vi "SbigOpen.vi"(2 "SbigDataList":cluster{"TagName":string, "Serial":string}[](array[cluster])=[{"TagName"="PI1-SBIG", "Serial"="01082913E_"}, {"TagName"="PI2-SBIG", "Serial"="02083139__"}], 9 "error in":errorcluster) -> (0 "Sbig Names out":string[](array[string])=["PI1-SBIG", "PI2-SBIG"], 6 "error out":errorcluster, 7 "Sbig infos":T1[](array[typedef])=[{"Readout modes number"=10, "Readout modes"=[{"Width"=765, "Height"=510, "Gain"=2.63, "pixelWidth"=9.0, "pixelHeight"=9.0}, {"Width"=382, "Height"=255, "Gain"=2.63, "pixelWidth"=18.0, "pixelHeight"=18.0}, {"Width"=255, "Height"=170, "Gain"=2.63, "pixelWidth"=27.0, "pixelHeight"=27.0}, {"Width"=765, "Height"=0, "Gain"=2.63, "pixelWidth"=9.0, "pixelHeight"=9.0}, {"Width"=382, "Height"=0, "Gain"=2.63, "pixelWidth"=18.0, "pixelHeight"=9.0}, {"Width"=255, "Height"=0, "Gain"=2.63, "pixelWidth"=27.0, "pixelHeight"=9.0}, {"Width"=765, "Height"=510, "Gain"=2.63, "pixelWidth"=9.0, "pixelHeight"=9.0}, {"Width"=382, "Height"=255, "Gain"=2.63, "pixelWidth"=18.0, "pixelHeight"=18.0}, {"Width"=255, "Height"=170, "Gain"=2.63, "pixelWidth"=27.0, "pixelHeight"=27.0}, {"Width"=85, "Height"=56, "Gain"=2.63, "pixelWidth"=81.0, "pixelHeight"=81.0}], "Handle"=[2]}, {"Readout modes number"=0, "Readout modes"=[], "Handle"=[]}])   [LabVIEW 2009]
uses:
  Controls/SbigReference.ctl
panel:
  out "Sbigs":string[](array[string])
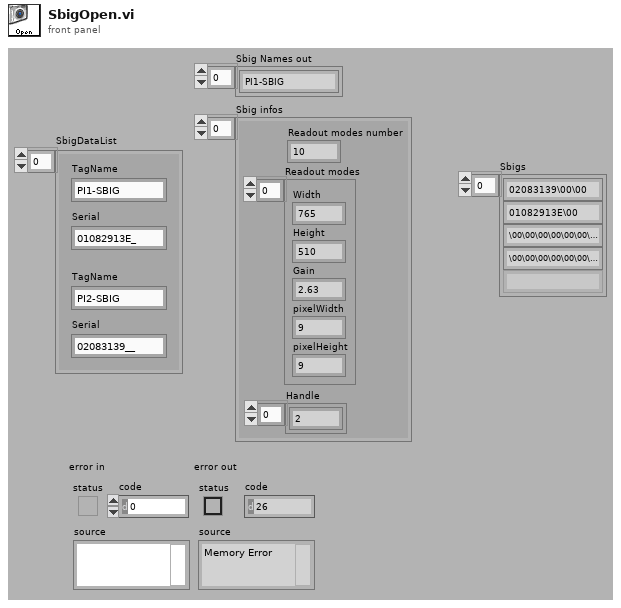
[diagram p1: front panel]
types:
  T1 = typedef "SbigReference.ctl" = cluster{"Readout modes number":u16, "Readout modes":cluster{"Width":u16, "Height":u16, "Gain":dbl, "pixelWidth":dbl, "pixelHeight":dbl}[], "Handle":u16[]}
  T2 = enum16{"0-NoCommand", "1-StartExposure", "2-EndExposure", "3-ReadoutLine", "4-DumpLines", "5-SetTemperatureRegulation", "6-QueryTemperatureStatus", "7-ActivateRelay", "8-PulseOut", "9-EstablishLink", "10-GetDriverInfo", "11-GetCCDInfo", "12-QueryCommandStatus", "13-MiscellaneousControl", "14-ReadSubstractLine", "15-UpdateClock", "16-ReadOffset", "17-OpenDriver", "18-CloseDriver", "19-TXSerialBytes", "20-GetSerialStatus", "21-AOTipTilt", "22-AOSetFocus", "23-AODelay", "24-GetTurboStatus", "25-EndReadout", "26-GetUSTimer", "27-OpenDevice", "28-CloseDevice", "29-SetIRQL", "30-GetIRQL", "31-GetLine", "32-GetLinkStatus", "33-GetDriverHandle", "34-SetDriverHandle", "35-StartReadout", "36-GetErrorString", "37-SetDriverControl", "38-GetDriverControl", "39-USBADControl", "40-QueryUSB", "41-GetPentiumCycleCount", "42-RWUSBI2C", "43-CFW"}
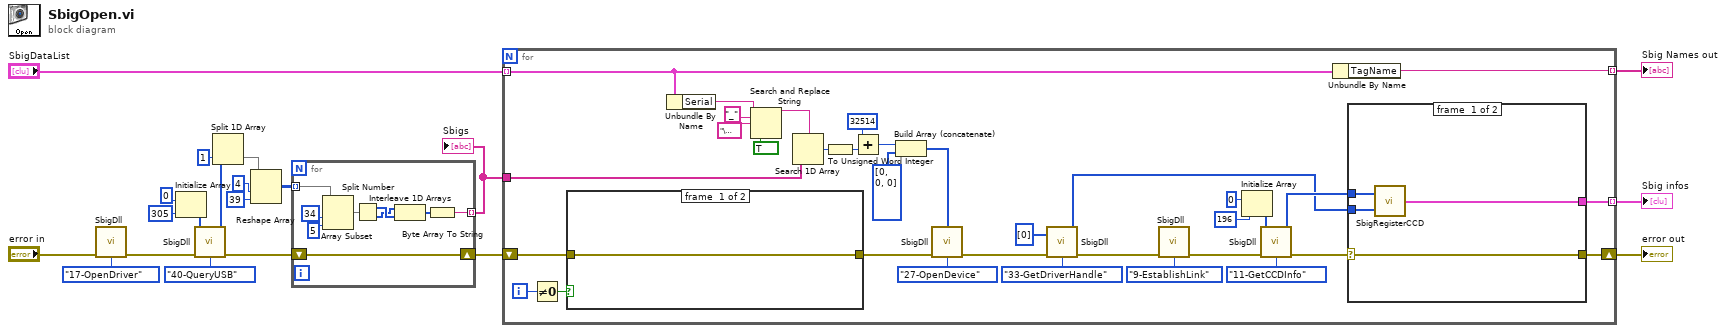
[diagram p0: block diagram]
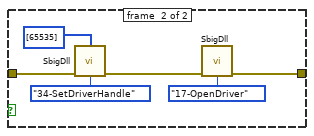
[diagram p2: hidden frame]
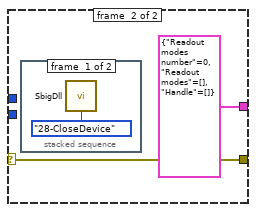
[diagram p3: hidden frame]
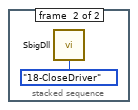
[diagram p4: hidden frame]
diagram:
  n1 = call "SbigDll.vi"("error in (no error)"="error in", "Command"=T2."17-OpenDriver") -> ("error out"=w6:errorcluster)  [unwired: 2 in, 3 out]
  n2 = Initialize Array(u16 0, 305 ("taille de la dimension")) -> (w5:u16[])
  n3 = call "SbigDll.vi"("error in (no error)"=w6, "Command"=T2."40-QueryUSB", "Results In"=w5) -> ("error out"=w15:errorcluster, "Results Out"=w13:u16[])  [unwired: 1 in, 2 out]
  n4 = Split 1D Array(array=w13, index=1 ("indice")) -> (second subarray=w14:u16[])  [unwired: 1 out]
  n5 = Reshape Array(w14, 4 ("taille de la dimension"), 39 ("taille de la dimension")) -> (w4:u16[][])
  n6 = for {
    shift-right: [w27] -> w3
    shift-left: w15 -> [w27]
    tunnel: [w28] -> w2 mode=indexing
    tunnel: w4 -> [w21] mode=indexing
    n7 = Array Subset(array=w21, index=34 ("indice"), length=5 ("longueur")) -> (w22:u16[])
    n8 = Split Number(x=w22) -> (hi(x)=w24:u8[], lo(x)=w23:u8[])
    n9 = Interleave 1D Arrays(w23, w24) -> (w29:u8[])
    n10 = Byte Array To String(unsigned byte array=w29) -> (string=w28:string)
  }
  "Sbigs" <- w2
  n11 = for {
    shift-right: [w53] -> w20
    shift-left: w3 -> [w36]
    tunnel: "SbigDataList" -> [w50] mode=indexing
    tunnel: [w52] -> w17 mode=indexing
    tunnel: [w49] -> w18 mode=indexing
    tunnel: w2 -> [w48]
    i -> [w38]
    n12 = Not Equal To 0?(x=w38) -> (x != 0?=w37:bool)
    n13 = case shown="True" w37 {
      tunnel: w36 -> [w64 w69]
      tunnel: [w64 w65] -> w35
      frame #0 {
      }
      frame #1 {
        n14 = call "SbigDll.vi"("error in (no error)"=w69, "Command"=T2."34-SetDriverHandle", "Parameters"=u16[] [65535] ("Results In")) -> ("error out"=w66:errorcluster)  [unwired: 1 in, 3 out]
        n15 = call "SbigDll.vi"("error in (no error)"=w66, "Command"=T2."17-OpenDriver") -> ("error out"=w65:errorcluster)  [unwired: 2 in, 3 out]
      }
    }
    n16 = Unbundle By Name(w50) -> ("Serial"=w51:string)
    n17 = Search and Replace String(replace all?=TRUE ("tout remplacer ? (F)"), input string=w51, search string="_" ("chaîne recherchée"), replace string="\u0000" ("chaîne de remplacement (\"\")")) -> (result string=w34:string)  [unwired: 1 in, 6 out]
    n18 = Search 1D Array(1D array=w48, element=w34) -> (index of element=w46:i32)  [unwired: 1 out]
    n19 = To Unsigned Word Integer(number=w46) -> (unsigned 16bit integer=w43:u16)
    n20 = Add(x=u16 32514, y=w43) -> (x+y=w45:u16)
    n21 = Build Array (concatenate)(w45, u16[] [0, 0, 0] ("Constante tableau")) -> (w39:u16[])
    n22 = call "SbigDll.vi"("error in (no error)"=w35, "Command"=T2."27-OpenDevice", "Parameters"=w39) -> ("error out"=w32:errorcluster)  [unwired: 1 in, 3 out]
    n23 = call "SbigDll.vi"("error in (no error)"=w32, "Command"=T2."33-GetDriverHandle", "Results In"=u16[] [0]) -> ("error out"=w31:errorcluster, "Results Out"=w30:u16[])  [unwired: 1 in, 2 out]
    n24 = call "SbigDll.vi"("error in (no error)"=w31, "Command"=T2."9-EstablishLink") -> ("error out"=w63:errorcluster)  [unwired: 2 in, 3 out]
    n25 = Initialize Array(u16 0, 196 ("Indice")) -> (w55:u16[])
    n26 = call "SbigDll.vi"("error in (no error)"=w63, "Command"=T2."11-GetCCDInfo", "Results In"=w55) -> ("error out"=w33:errorcluster, "Results Out"=w54:u16[])  [unwired: 1 in, 2 out]
    n27 = Unbundle By Name(w50) -> ("TagName"=w49:string)
    n28 = case shown="No Error" w33 {
      selector: w33 -> [w72 w76]
      tunnel: [w72 w76] -> w53
      tunnel: w54 -> [w74 _]
      tunnel: [w73 T1 {"Readout modes number"=0, "Readout modes"=[], "Handle"=[]} ("CCD")] -> w52
      tunnel: w30 -> [w71 _]
      frame #0 {
        n29 = call "SbigRegisterCCD.vi"("GetDriverHandle"=w71, "GetCCDInfo"=w74) -> ("CCD"=w73:T1)
      }
      frame #1 {
        n30 = stacked-sequence {
          frame #0 {
            n31 = call "SbigDll.vi"("Command"=T2."28-CloseDevice") -> ()  [unwired: 3 in, 4 out]
          }
          frame #1 {
            n32 = call "SbigDll.vi"("Command"=T2."18-CloseDriver") -> ()  [unwired: 3 in, 4 out]
          }
        }
      }
    }
  }
  "error out" <- w20
  "Sbig Names out" <- w18
  "Sbig infos" <- w17
